vi "Calculate Velocity and PV.vi"(11 "Acceleration Array":dbl[](array[numeric])) -> (0 "Peak velocity":dbl, 1 "Velocity Array":dbl[](array[numeric]))   [LabVIEW 2016]
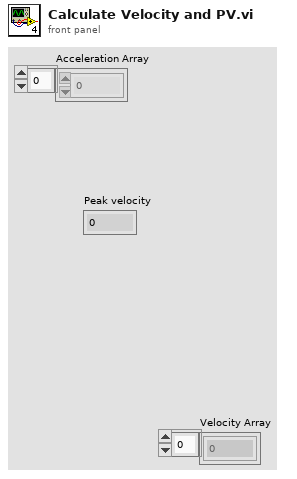
[diagram p1: front panel]
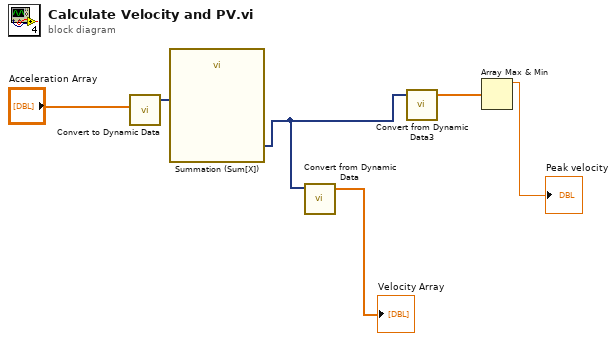
[diagram p0: block diagram]
diagram:
  n1 = call "Convert to Dynamic Data"("Array"="Acceleration Array") -> ("Dynamic Data Type"=w4:dynamicdata)  [unwired: 3 in]
  n2 = call "Summation (Sum[X])"("Signals"=w4) -> ("Result"=w3:dynamicdata)  [unwired: 1 in, 5 out]
  n3 = call "Convert from Dynamic Data"("Dynamic Data Type"=w3) -> ("Array"=→"Velocity Array":dbl[])  [unwired: 3 in]
  n4 = call "Convert from Dynamic Data3"("Dynamic Data Type"=w3) -> ("Array"=w2:dbl[])  [unwired: 3 in]
  n5 = Array Max & Min(array=w2) -> (max value=→"Peak velocity":dbl)  [unwired: 3 out]
